vi "CreateCommands.vi"   [LabVIEW 2015]
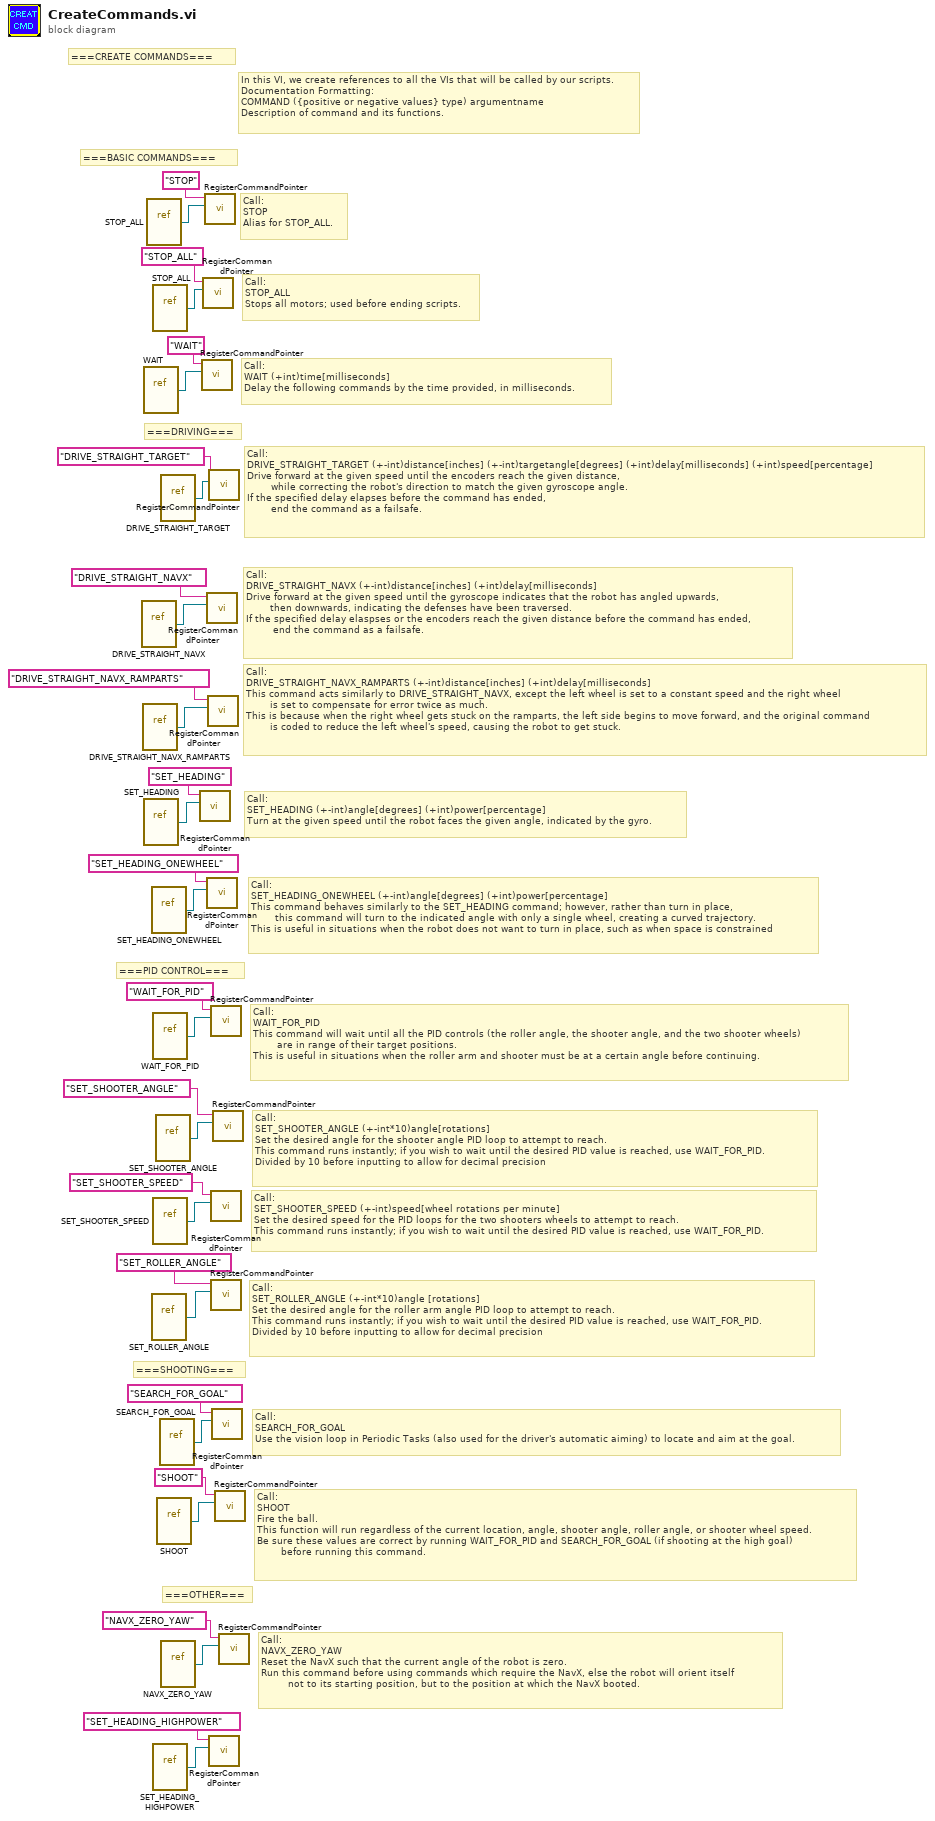
[diagram p0: block diagram]
diagram:
  # "===CREATE COMMANDS==="
  # "In this VI, we create references to all the VIs that will be called by our scripts.\nDocumentation Formatting:\nCOMMAND ({positive or negative values} type) argumentname\nDescription of command and its functions."
  # "===OTHER==="
  # "===SHOOTING==="
  # "===PID CONTROL==="
  # "===DRIVING==="
  # "===BASIC COMMANDS==="
  # "Call:\nSET_ROLLER_ANGLE (+-int*10)angle [rotations]\nSet the desired angle for the roller arm angle PID loop to attempt to reach.\nThis command runs instantly; if you wish to wait until the desired PID value is reached, use WAIT_FOR_PID.\nDivided by 10 before inputting to allow for decimal precision"
  # "Call:\nDRIVE_STRAIGHT_NAVX_RAMPARTS (+-int)distance[inches] (+int)delay[milliseconds]\nThis command acts similarly to DRIVE_STRAIGHT_NAVX, except the left wheel is set to a constant speed and the right wheel\n        is set to compensate for error twice as much.\nThis is because when the right wheel gets stuck on the ramparts, the left side begins to move forward, and the original command\n        is coded to reduce the left wheel's speed, causing the robot to get stuck."
  # "Call:\nNAVX_ZERO_YAW\nReset the NavX such that the current angle of the robot is zero.\nRun this command before using commands which require the NavX, else the robot will orient itself\n         not to its starting position, but to the position at which the NavX booted."
  # "Call:\nDRIVE_STRAIGHT_TARGET (+-int)distance[inches] (+-int)targetangle[degrees] (+int)delay[milliseconds] (+int)speed[percentage]\nDrive forward at the given speed until the encoders reach the given distance,\n        while correcting the robot's direction to match the given gyroscope angle.\nIf the specified delay elapses before the command has ended,\n        end the command as a failsafe."
  # "Call:\nSHOOT\nFire the ball.\nThis function will run regardless of the current location, angle, shooter angle, roller angle, or shooter wheel speed.\nBe sure these values are correct by running WAIT_FOR_PID and SEARCH_FOR_GOAL (if shooting at the high goal)\n        before running this command."
  # "Call:\nSET_SHOOTER_SPEED (+-int)speed[wheel rotations per minute]\nSet the desired speed for the PID loops for the two shooters wheels to attempt to reach.\nThis command runs instantly; if you wish to wait until the desired PID value is reached, use WAIT_FOR_PID."
  # "Call:\nWAIT_FOR_PID\nThis command will wait until all the PID controls (the roller angle, the shooter angle, and the two shooter wheels)\n        are in range of their target positions.\nThis is useful in situations when the roller arm and shooter must be at a certain angle before continuing."
  # "Call:\nSET_HEADING (+-int)angle[degrees] (+int)power[percentage]\nTurn at the given speed until the robot faces the given angle, indicated by the gyro."
  # "Call:\nSET_SHOOTER_ANGLE (+-int*10)angle[rotations]\nSet the desired angle for the shooter angle PID loop to attempt to reach.\nThis command runs instantly; if you wish to wait until the desired PID value is reached, use WAIT_FOR_PID.\nDivided by 10 before inputting to allow for decimal precision"
  # "Call:\nSET_HEADING_ONEWHEEL (+-int)angle[degrees] (+int)power[percentage]\nThis command behaves similarly to the SET_HEADING command; however, rather than turn in place,\n        this command will turn to the indicated angle with only a single wheel, creating a curved trajectory.\nThis is useful in situations when the robot does not want to turn in place, such as when space is constrained"
  # "Call:\nSEARCH_FOR_GOAL\nUse the vision loop in Periodic Tasks (also used for the driver's automatic aiming) to locate and aim at the goal."
  # "Call:\nSTOP\nAlias for STOP_ALL."
  # "Call:\nSTOP_ALL\nStops all motors; used before ending scripts."
  # "Call:\nDRIVE_STRAIGHT_NAVX (+-int)distance[inches] (+int)delay[milliseconds]\nDrive forward at the given speed until the gyroscope indicates that the robot has angled upwards,\n        then downwards, indicating the defenses have been traversed.\nIf the specified delay elaspses or the encoders reach the given distance before the command has ended,\n         end the command as a failsafe."
  # "Call:\nWAIT (+int)time[milliseconds]\nDelay the following commands by the time provided, in milliseconds."
  n1 = vi-ref "DRIVE_STRAIGHT_NAVX.vi"() -> (w21:refnum<vi>)
  n2 = vi-ref "DRIVE_STRAIGHT_NAVX_RAMPARTS.vi"() -> (w3:refnum<vi>)
  n3 = vi-ref "WAIT.vi"() -> (w29:refnum<vi>)
  n4 = vi-ref "SET_HEADING.vi"() -> (w25:refnum<vi>)
  n5 = vi-ref "STOP_ALL.vi"() -> (w28:refnum<vi>)
  n6 = vi-ref "SET_HEADING_ONEWHEEL.vi"() -> (w17:refnum<vi>)
  n7 = vi-ref "SET_ROLLER_ANGLE.vi"() -> (w19:refnum<vi>)
  n8 = vi-ref "STOP_ALL.vi"() -> (w31:refnum<vi>)
  n9 = vi-ref "WAIT_FOR_PID.vi"() -> (w13:refnum<vi>)
  n10 = vi-ref "SET_SHOOTER_SPEED.vi"() -> (w11:refnum<vi>)
  n11 = vi-ref "SET_HEADING_HIGHPOWER.vi"() -> (w1:refnum<vi>)
  n12 = vi-ref "SET_SHOOTER_ANGLE.vi"() -> (w15:refnum<vi>)
  n13 = vi-ref "SHOOT.vi"() -> (w10:refnum<vi>)
  n14 = vi-ref "SEARCH_FOR_GOAL.vi"() -> (w23:refnum<vi>)
  n15 = vi-ref "DRIVE_STRAIGHT_TARGET.vi"() -> (w7:refnum<vi>)
  n16 = vi-ref "NAVX_ZERO_YAW.vi"() -> (w6:refnum<vi>)
  n17 = call "RegisterCommandPointer.vi"("Strict-Typed VI Refnum"=w25, "Name"="SET_HEADING") -> ()  [unwired: 10 in]
  n18 = call "RegisterCommandPointer.vi"("Strict-Typed VI Refnum"=w29, "Name"="WAIT") -> ()  [unwired: 10 in]
  n19 = call "RegisterCommandPointer.vi"("Strict-Typed VI Refnum"=w31, "Name"="STOP_ALL") -> ()  [unwired: 10 in]
  n20 = call "RegisterCommandPointer.vi"("Strict-Typed VI Refnum"=w28, "Name"="STOP") -> ()  [unwired: 10 in]
  n21 = call "RegisterCommandPointer.vi"("Strict-Typed VI Refnum"=w21, "Name"="DRIVE_STRAIGHT_NAVX") -> ()  [unwired: 10 in]
  n22 = call "RegisterCommandPointer.vi"("Strict-Typed VI Refnum"=w17, "Name"="SET_HEADING_ONEWHEEL") -> ()  [unwired: 10 in]
  n23 = call "RegisterCommandPointer.vi"("Strict-Typed VI Refnum"=w3, "Name"="DRIVE_STRAIGHT_NAVX_RAMPARTS") -> ()  [unwired: 10 in]
  n24 = call "RegisterCommandPointer.vi"("Strict-Typed VI Refnum"=w7, "Name"="DRIVE_STRAIGHT_TARGET") -> ()  [unwired: 10 in]
  n25 = call "RegisterCommandPointer.vi"("Strict-Typed VI Refnum"=w1, "Name"="SET_HEADING_HIGHPOWER") -> ()  [unwired: 10 in]
  n26 = call "RegisterCommandPointer.vi"("Strict-Typed VI Refnum"=w13, "Name"="WAIT_FOR_PID") -> ()  [unwired: 10 in]
  n27 = call "RegisterCommandPointer.vi"("Strict-Typed VI Refnum"=w11, "Name"="SET_SHOOTER_SPEED") -> ()  [unwired: 10 in]
  n28 = call "RegisterCommandPointer.vi"("Strict-Typed VI Refnum"=w19, "Name"="SET_ROLLER_ANGLE") -> ()  [unwired: 10 in]
  n29 = call "RegisterCommandPointer.vi"("Strict-Typed VI Refnum"=w23, "Name"="SEARCH_FOR_GOAL") -> ()  [unwired: 10 in]
  n30 = call "RegisterCommandPointer.vi"("Strict-Typed VI Refnum"=w15, "Name"="SET_SHOOTER_ANGLE") -> ()  [unwired: 10 in]
  n31 = call "RegisterCommandPointer.vi"("Strict-Typed VI Refnum"=w10, "Name"="SHOOT") -> ()  [unwired: 10 in]
  n32 = call "RegisterCommandPointer.vi"("Strict-Typed VI Refnum"=w6, "Name"="NAVX_ZERO_YAW") -> ()  [unwired: 10 in]
